vi "Accumulated Correlation HPRF.vi"(5 "Ntheta":i32=16, 6 "Sensor Locations (cm)":dbl[][](array[numeric])=[[0.0, 0.0, -5.08], [11.43, 0.0, 0.0], [0.0, 11.43, 0.0], [-11.43, 0.0, 0.0], [0.0, -11.43, 0.0], [0.0, 0.0, 5.08]], 7 "Nr":i32=16, 8 "Sound Velocity (cm/s)":dbl=576000.0, 9 "Sampling Rate":i32=500000, 11 "Waveforms":dbl[][](array[numeric])) -> (2 "Coordinates (m)":cluster{"x":dbl, "y":dbl, "z":dbl})   [LabVIEW 2013]
uses:
  <vilib>/Analysis/2dsp.llb/1D Cross Correlation (DBL).vi
  <vilib>/Analysis/NI_AALPro.lvlib
panel:
  out "Signals":dbl[][](graph)
  out "output variable 3":dbl
  out "output variable 2":dbl
  out "output variable":dbl
  out "subarray 2":dbl[][](array[numeric])
  out "subarray":dbl[][](array[numeric])
  out "size(s)":i32[](array[numeric])
  out "theta":dbl
  out "r":dbl
  out "Correlation":dbl[][](graph)
  out "Lag Matrix":dbl[][](array[numeric])
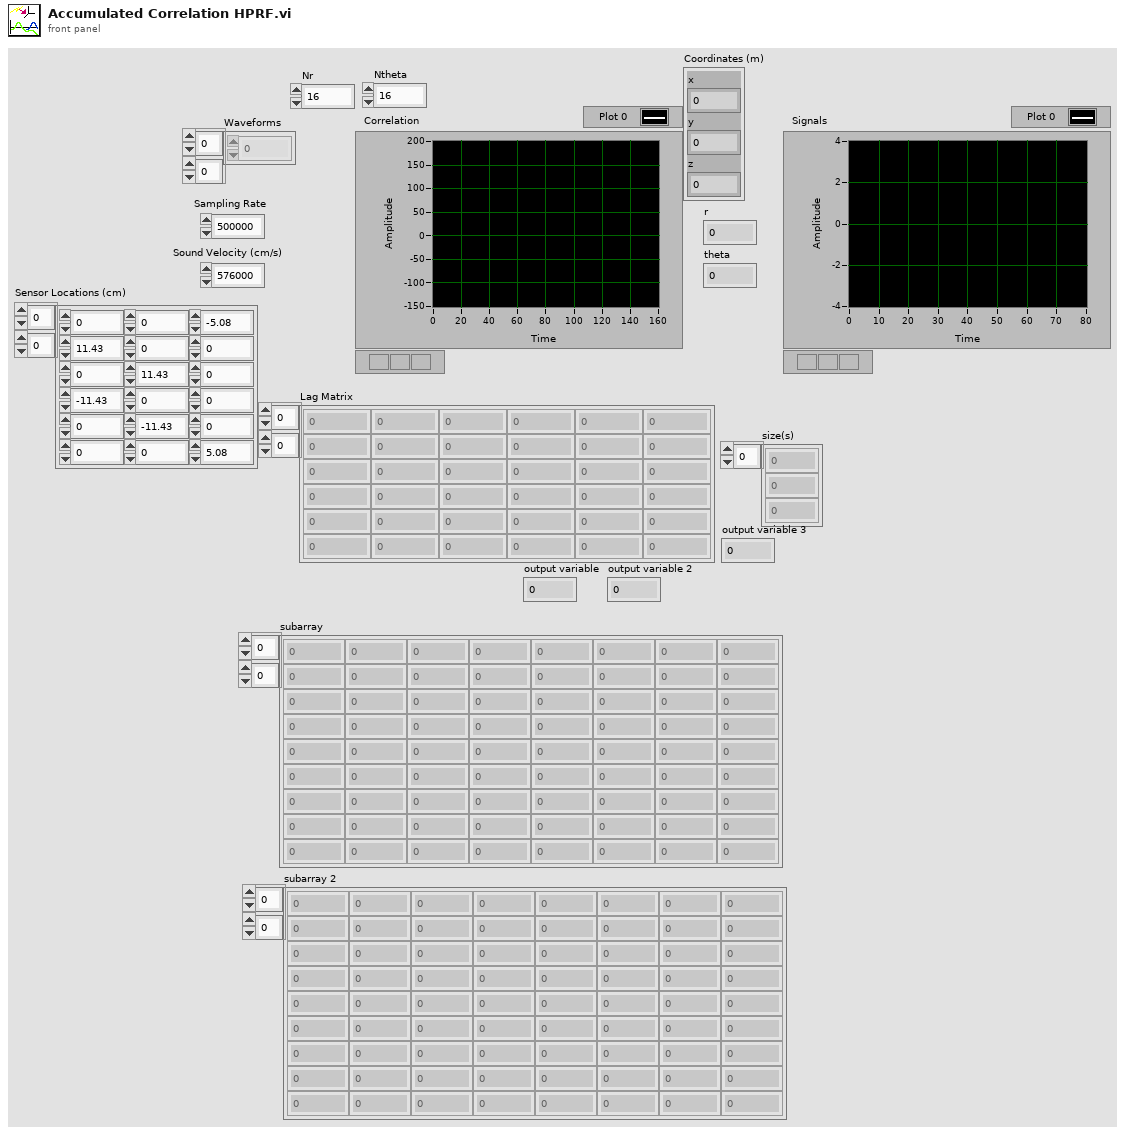
[diagram p1: front panel]
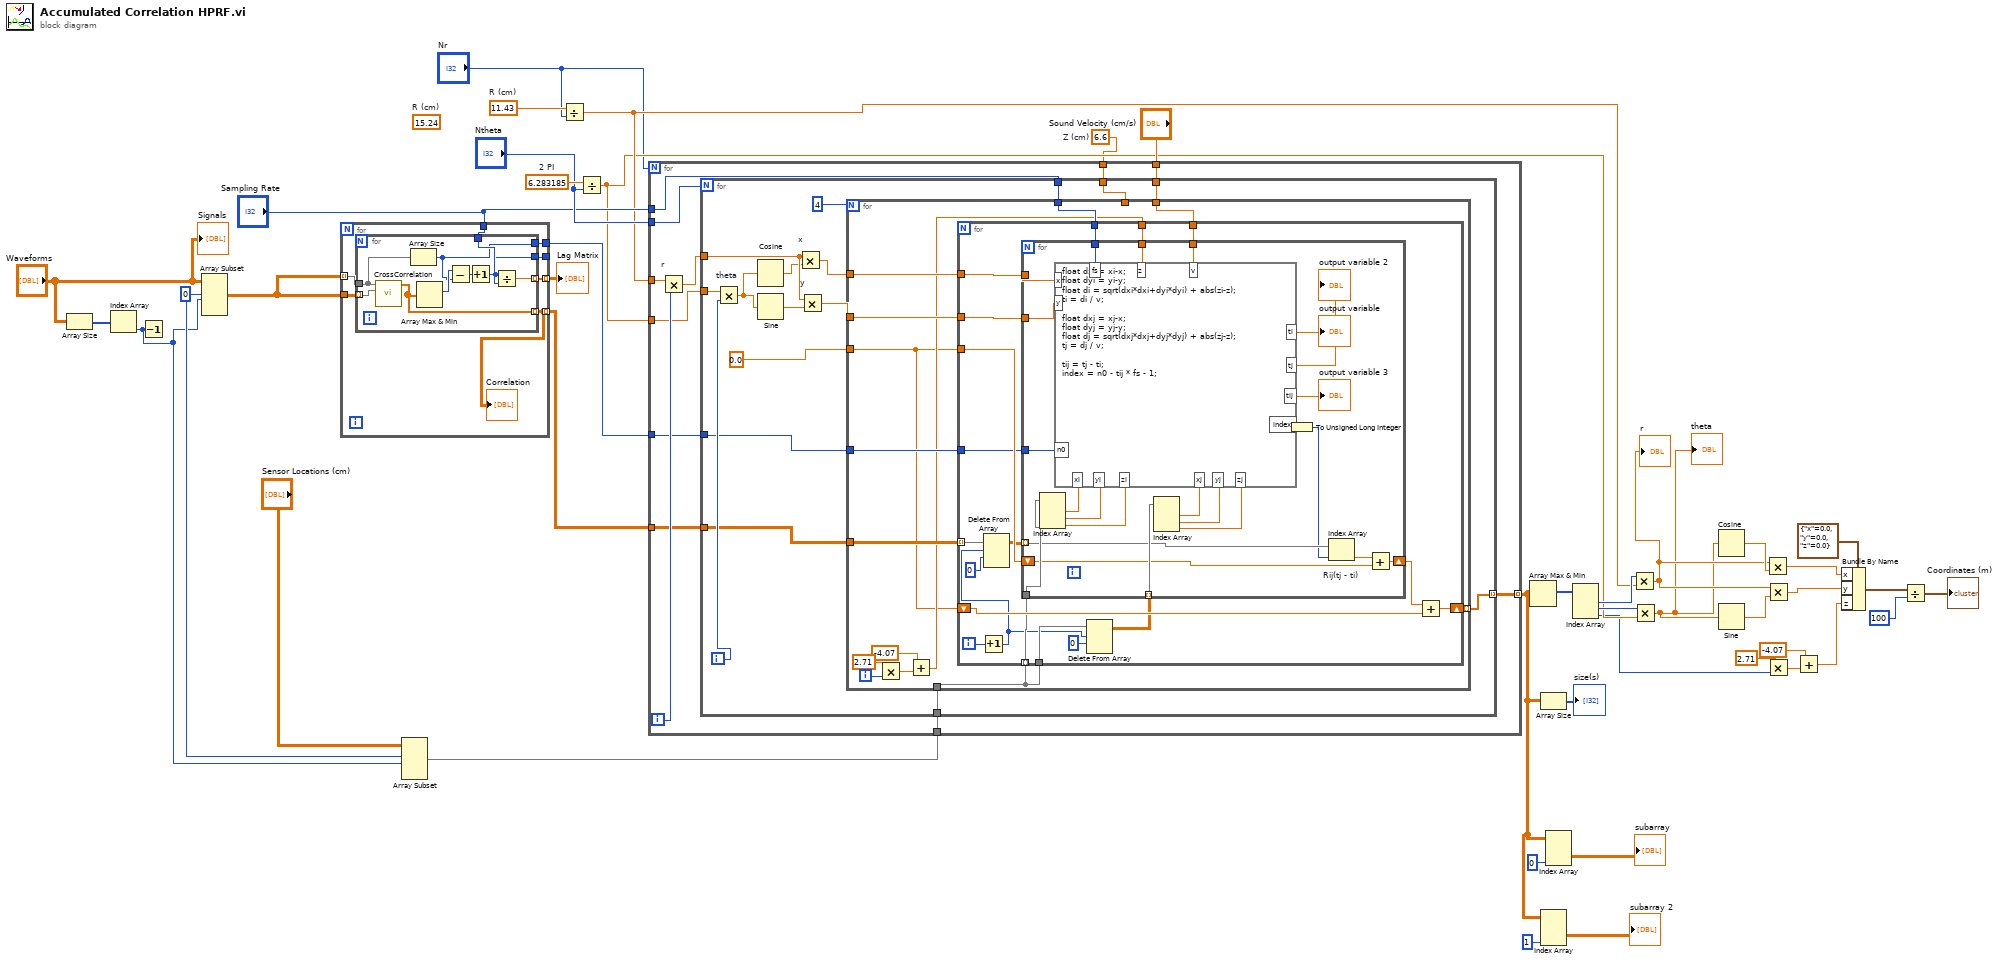
[diagram p0: block diagram]
diagram:
  (unwired) 15.24  # R (cm)
  w19 = 0 ("index")
  w42 = 11.43  # R (cm)
  w41 = 6.283185  # 2 PI
  w17 = 6.6  # Z (cm)
  n1 = Array Size(array="Waveforms") -> (size(s)=w4:i32[])
  n2 = Index Array(array=w4) -> (element=w2:i32)  [unwired: 1 in]
  n3 = Decrement(x=w2) -> ()  [unwired: 1 out]
  n4 = Array Subset(array="Waveforms", index (row)=w19, length (row)=w2) -> (w21:dbl[][])  [unwired: 2 in]
  n5 = for {
    tunnel: w21 -> [w49] mode=indexing
    tunnel: w21 -> [w50]
    tunnel: "Sampling Rate" -> [w48]
    tunnel: [w47] -> w43 mode=indexing
    tunnel: [w45] -> w37 mode=indexing
    tunnel: [w46] -> _
    tunnel: [w44] -> w1
    n6 = for {
      tunnel: w50 -> [w59] mode=indexing
      tunnel: w49 -> [w58]
      tunnel: w48 -> [w57]
      tunnel: [w56] -> w47 mode=indexing
      tunnel: [w53] -> w45 mode=indexing
      tunnel: [w54] -> w46
      tunnel: [w51] -> w44
      n7 = call-poly <vilib>:"CrossCorrelation.vi"("Y"=w59, "X"=w58) -> ("Rxy"=w53:dbl[])  [unwired: 8 in, 1 out]
      n8 = Array Size(array=w58) -> (size(s)=w51:i32)
      n9 = Array Max & Min(array=w53) -> (max index (indices)=w52:i32)  [unwired: 3 out]
      n10 = Subtract(x=w52, y=w51) -> (x-y=w55:i32)
      n11 = Increment(x=w55) -> (x+1=w54:i32)
      n12 = Divide(x=w54, y=w57) -> (x/y=w56:dbl)
    }
    "Correlation" <- w45
  }
  "Lag Matrix" <- w43
  n13 = Array Subset(array="Sensor Locations (cm)", index (row)=w19, length (row)=w2) -> (w5:dbl[][])  [unwired: 2 in]
  n14 = Divide(x=w42, y="Nr") -> (x/y=w33:dbl)
  n15 = Divide(x=w41, y="Ntheta") -> (x/y=w32:dbl)
  n16 = for {
    N: "Nr" -> [_]
    tunnel: [w71] -> w6 mode=indexing
    tunnel: "Ntheta" -> [w70]
    tunnel: w33 -> [w69]
    tunnel: w32 -> [w67]
    tunnel: w5 -> [w66]
    tunnel: w17 -> [w65]
    tunnel: "Sound Velocity (cm/s)" -> [w64]
    tunnel: "Sampling Rate" -> [w63]
    tunnel: w1 -> [w62]
    tunnel: w37 -> [w61]
    i -> [w68]
    n17 = Multiply "r"(x=w69, y=w68) -> (x*y=w60:dbl)
    n18 = for {
      N: w70 -> [_]
      tunnel: [w87] -> w71 mode=indexing
      tunnel: w67 -> [w86]
      tunnel: w60 -> [w84]
      tunnel: w66 -> [w81]
      tunnel: w65 -> [w73]
      tunnel: w64 -> [w80]
      tunnel: w63 -> [w79]
      tunnel: w62 -> [w78]
      tunnel: w61 -> [w77]
      i -> [w85]
      n19 = Multiply "theta"(x=w86, y=w85) -> (x*y=w76:dbl)
      n20 = Cosine(x=w76) -> (cos(x)=w83:dbl)
      n21 = Sine(x=w76) -> (sin(x)=w82:dbl)
      n22 = Multiply "x"(x=w84, y=w83) -> (x*y=w75:dbl)
      n23 = Multiply "y"(x=w84, y=w82) -> (x*y=w74:dbl)
      n24 = for {
        N: 4 -> [_]
        tunnel: 0.0 -> [w89]
        tunnel: [w102] -> w87 mode=indexing
        tunnel: w81 -> [w101]
        tunnel: w80 -> [w100]
        tunnel: w79 -> [w99]
        tunnel: w78 -> [w98]
        tunnel: w77 -> [w97]
        tunnel: w75 -> [w96]
        tunnel: w74 -> [w95]
        tunnel: w73 -> [_]
        i -> [w94]
        n25 = Multiply(x=2.71, y=w94) -> (x*y=w92:dbl)
        n26 = Add(x=-4.07, y=w92) -> (x+y=w90:dbl)
        n27 = for {
          shift-right: [w118] -> w102
          shift-left: w89 -> [w119]
          tunnel: w89 -> [w121]
          tunnel: w96 -> [w117]
          tunnel: w95 -> [w116]
          tunnel: w101 -> [w115] mode=indexing
          tunnel: w101 -> [w109]
          tunnel: w90 -> [w114]
          tunnel: w100 -> [w113]
          tunnel: w99 -> [w112]
          tunnel: w98 -> [w111]
          tunnel: w97 -> [w106] mode=indexing
          i -> [w110]
          n28 = Increment(x=w110) -> (x+1=w103:i32)
          n29 = Delete From Array(array=w106, length=w103, index (row)=0) -> (array with subset deleted=w105:dbl[][])  [unwired: 1 in, 1 out]
          n30 = Delete From Array(array=w109, length=w103, index (row)=0) -> (array with subset deleted=w107:dbl[][])  [unwired: 1 in, 1 out]
          n31 = for {
            shift-right: [w129] -> w120
            shift-left: w121 -> [w127]
            tunnel: w117 -> [w140]
            tunnel: w116 -> [w139]
            tunnel: w107 -> [w143] mode=indexing
            tunnel: w115 -> [w144]
            tunnel: w114 -> [w142]
            tunnel: w113 -> [w141]
            tunnel: w112 -> [w134]
            tunnel: w111 -> [w133]
            tunnel: w105 -> [w131] mode=indexing
            n32 = Index Array(array=w144) -> (element #1=w138:dbl, element #2=w137:dbl, element #3=w126:dbl)  [unwired: 3 in]
            n33 = Index Array(array=w143) -> (element #1=w136:dbl, element #2=w135:dbl, element #3=w125:dbl)  [unwired: 3 in]
            n34 = formula code="float dxi = xi-x;\nfloat dyi = yi-y;\nfloat di = sqrt(dxi*dxi+dyi*dyi) + abs(zi-z);\nti = di / v;\n\nfloat dxj = xj-x;\nfloat dyj = yj-y;\nfloat dj = sqrt(dxj*dxj+dyj*dyj) + abs(zj-z);\ntj = dj / v;\n\ntij = tj - ti;\nindex = n0 - tij * fs - 1;"("xi"=w138, "yi"=w137, "xj"=w136, "yj"=w135, "x"=w140, "y"=w139, "z"=w142, "v"=w141, "fs"=w134, "n0"=w133, "zi"=w126, "zj"=w125) -> ("index"=w132:dbl, "ti"=→"output variable":dbl, "tj"=→"output variable 2":dbl, "tij"=→"output variable 3":dbl)
            n35 = To Unsigned Long Integer(number=w132) -> (unsigned 32bit integer=w130:u32)
            n36 = Index Array "Rij(tj - ti)"(array=w131, index=w130) -> (element=w128:dbl)
            n37 = Add(x=w128, y=w127) -> (x+y=w129:dbl)
          }
          n38 = Add(x=w120, y=w119) -> (x+y=w118:dbl)
        }
      }
    }
  }
  n39 = Array Max & Min(array=w6) -> (max index (indices)=w36:i32[])  [unwired: 3 out]
  n40 = Array Size(array=w6) -> (size(s)=→"size(s)":i32[])
  n41 = Index Array(array=w6, index (dim 2)=1 ("disabled index (col)")) -> (element=→"subarray 2":dbl[][])  [unwired: 2 in]
  n42 = Index Array(array=w6, index (dim 2)=0 ("disabled index (col)")) -> (element=→"subarray":dbl[][])  [unwired: 2 in]
  n43 = Index Array(array=w36) -> (element #1=w35:i32, element #2=w34:i32, element #3=w13:i32)  [unwired: 3 in]
  n44 = Multiply(x=w35, y=w33) -> (x*y=w29:dbl)
  "r" <- w29
  n45 = Multiply(x=w34, y=w32) -> (x*y=w28:dbl)
  "theta" <- w28
  n46 = Cosine(x=w28) -> (cos(x)=w31:dbl)
  n47 = Sine(x=w28) -> (sin(x)=w30:dbl)
  n48 = Multiply ("x*y")(x=w29, y=w31) -> (x*y=w27:dbl)
  n49 = Multiply ("x*y")(x=w29, y=w30) -> (x*y=w26:dbl)
  n50 = Multiply(x=2.71, y=w13) -> (x*y=w15:dbl)
  n51 = Add(x=-4.07, y=w15) -> (x+y=w12:dbl)
  n52 = Bundle By Name(cluster=cluster{"x":dbl, "y":dbl, "z":dbl} {"x"=0.0, "y"=0.0, "z"=0.0} ("input cluster"), "x"=w27, "y"=w26, "z"=w12) -> (w24:cluster{"x":dbl, "y":dbl, "z":dbl})
  n53 = Divide(x=w24, y=100 ("index (row)")) -> (x/y=→"Coordinates (m)":cluster{"x":dbl, "y":dbl, "z":dbl})
  "Signals" <- "Waveforms"
